vi "nanocal -- nuclear schottky goodness V3.vi"(7 "weighting strategy":T1, 8 "dz/dω IN (V)":cdb[](array[numeric])=[1.7183506006211996e-05+0.0i, 1.7124360968751133e-05+0.0i, 1.7049104347380084e-05+0.0i, 1.700437896335042e-05+0.0i, 1.6984579723285106e-05+0.0i, 1.702277369054923e-05+0.0i, 1.713094025845651e-05+0.0i, 1.734249707866828e-05+0.0i, 1.768320429215342e-05+0.0i, 1.8195281152538477e-05+0.0i, 1.8917228661806973e-05+0.0i, 1.9897834564883332e-05+0.0i, 2.154104046962704e-05+0.0i, 2.3247799321765792e-05+0.0i, 2.5364678450551808e-05+0.0i, 2.8645788781885885e-05+0.0i, 3.204749554800641e-05+0.0i, 3.783559691555022e-05+0.0i, 4.245015867332296e-05+0.0i, 4.909131821431355e-05+0.0i, 5.511821898441184e-05+0.0i, 6.178843506022867e-05+0.0i, 7.1079604965352e-05+0.0i, 7.922304381453334e-05+0.0i, 8.814778883893872e-05+0.0i, 9.806709148886077e-05+0.0i, 0.00011119043245647465+0.0i, 0.00012253184919712196+0.0i, 0.00013777724317049346+0.0i, 0.0001508081004573332+0.0i, 0.00016547294918783876+0.0i, 0.00018003847596605868+0.0i, 0.00019518361086534857+0.0i, 0.00021134179818259658+0.0i, 0.0002372041782935464+0.0i, 0.00025518143132024254+0.0i, 0.0002835129702467886+0.0i, 0.0003060118087631287+0.0i, 0.00032860772064336976+0.0i, 0.0003492674091322389+0.0i, 0.00037498324855458583+0.0i, 0.00040021078021115026+0.0i, 0.00041969942568205823+0.0i, 0.00044367338947118773+0.0i, 0.0004634793607238068+0.0i, 0.00047921028781215815+0.0i, 0.0004880906353641744+0.0i, 0.0004932212623741357+0.0i, 0.000491476456593048+0.0i, 0.000480893803992059+0.0i, 0.0004535995818650303+0.0i, 0.000417087772881063+0.0i, 0.0003564148692854789+0.0i, 0.0003049201646356487+0.0i, 0.00021260191240459413+0.0i, 0.00011714858948470126+0.0i, 1.675457544365132e-05+0.0i, -6.8674075405897e-05+0.0i, -0.000156473047607305+0.0i, -0.00026709373934749337+0.0i, -0.0003544271565676041+0.0i, -0.00047937600197311275+0.0i, -0.0006086290582260493+0.0i, -0.0007031877411848573+0.0i, -0.0007564526901441745+0.0i, -0.000802489180995596+0.0i, -0.0008414596018105983+0.0i, -0.0008809346482248761+0.0i, -0.0009073902840241921+0.0i, -0.0009264953054508651+0.0i, -0.0009405659412141811+0.0i, -0.000951649722530156+0.0i, -0.0009557485581057351+0.0i, -0.0009558464741053665+0.0i, -0.0009509110176922098+0.0i, -0.0009411315169847015+0.0i, -0.0009303400913929496+0.0i, -0.0009171113529290538+0.0i, -0.0009022111527275027+0.0i, -0.0008813746494947608+0.0i, -0.0008581837971946129+0.0i, -0.0008372063466683705+0.0i, -0.0008165626610594428+0.0i, -0.0007901155435838691+0.0i, -0.0007682834352800848+0.0i, -0.000746231015527196+0.0i, -0.0007238798463130141+0.0i, -0.0007015567569177018+0.0i, -0.000679301954671598+0.0i, -0.0006572001413831251+0.0i, -0.000629855254567978+0.0i, -0.0006083942229188815+0.0i, -0.0005768631156754208+0.0i, -0.0005562177438951648+0.0i, -0.0005359092039599222+0.0i, -0.0005145186443378148+0.0i, -0.0004951602053444319+0.0i, -0.00047624970229075174+0.0i, -0.0004577401041527736+0.0i, -0.00043519037796120065+0.0i], 9 "Voltage IN (V)":cdb[](array[numeric])=[1.7183506006211996e-05+0.0i, 1.7124360968751133e-05+0.0i, 1.7049104347380084e-05+0.0i, 1.700437896335042e-05+0.0i, 1.6984579723285106e-05+0.0i, 1.702277369054923e-05+0.0i, 1.713094025845651e-05+0.0i, 1.734249707866828e-05+0.0i, 1.768320429215342e-05+0.0i, 1.8195281152538477e-05+0.0i, 1.8917228661806973e-05+0.0i, 1.9897834564883332e-05+0.0i, 2.154104046962704e-05+0.0i, 2.3247799321765792e-05+0.0i, 2.5364678450551808e-05+0.0i, 2.8645788781885885e-05+0.0i, 3.204749554800641e-05+0.0i, 3.783559691555022e-05+0.0i, 4.245015867332296e-05+0.0i, 4.909131821431355e-05+0.0i, 5.511821898441184e-05+0.0i, 6.178843506022867e-05+0.0i, 7.1079604965352e-05+0.0i, 7.922304381453334e-05+0.0i, 8.814778883893872e-05+0.0i, 9.806709148886077e-05+0.0i, 0.00011119043245647465+0.0i, 0.00012253184919712196+0.0i, 0.00013777724317049346+0.0i, 0.0001508081004573332+0.0i, 0.00016547294918783876+0.0i, 0.00018003847596605868+0.0i, 0.00019518361086534857+0.0i, 0.00021134179818259658+0.0i, 0.0002372041782935464+0.0i, 0.00025518143132024254+0.0i, 0.0002835129702467886+0.0i, 0.0003060118087631287+0.0i, 0.00032860772064336976+0.0i, 0.0003492674091322389+0.0i, 0.00037498324855458583+0.0i, 0.00040021078021115026+0.0i, 0.00041969942568205823+0.0i, 0.00044367338947118773+0.0i, 0.0004634793607238068+0.0i, 0.00047921028781215815+0.0i, 0.0004880906353641744+0.0i, 0.0004932212623741357+0.0i, 0.000491476456593048+0.0i, 0.000480893803992059+0.0i, 0.0004535995818650303+0.0i, 0.000417087772881063+0.0i, 0.0003564148692854789+0.0i, 0.0003049201646356487+0.0i, 0.00021260191240459413+0.0i, 0.00011714858948470126+0.0i, 1.675457544365132e-05+0.0i, -6.8674075405897e-05+0.0i, -0.000156473047607305+0.0i, -0.00026709373934749337+0.0i, -0.0003544271565676041+0.0i, -0.00047937600197311275+0.0i, -0.0006086290582260493+0.0i, -0.0007031877411848573+0.0i, -0.0007564526901441745+0.0i, -0.000802489180995596+0.0i, -0.0008414596018105983+0.0i, -0.0008809346482248761+0.0i, -0.0009073902840241921+0.0i, -0.0009264953054508651+0.0i, -0.0009405659412141811+0.0i, -0.000951649722530156+0.0i, -0.0009557485581057351+0.0i, -0.0009558464741053665+0.0i, -0.0009509110176922098+0.0i, -0.0009411315169847015+0.0i, -0.0009303400913929496+0.0i, -0.0009171113529290538+0.0i, -0.0009022111527275027+0.0i, -0.0008813746494947608+0.0i, -0.0008581837971946129+0.0i, -0.0008372063466683705+0.0i, -0.0008165626610594428+0.0i, -0.0007901155435838691+0.0i, -0.0007682834352800848+0.0i, -0.000746231015527196+0.0i, -0.0007238798463130141+0.0i, -0.0007015567569177018+0.0i, -0.000679301954671598+0.0i, -0.0006572001413831251+0.0i, -0.000629855254567978+0.0i, -0.0006083942229188815+0.0i, -0.0005768631156754208+0.0i, -0.0005562177438951648+0.0i, -0.0005359092039599222+0.0i, -0.0005145186443378148+0.0i, -0.0004951602053444319+0.0i, -0.00047624970229075174+0.0i, -0.0004577401041527736+0.0i, -0.00043519037796120065+0.0i], 10 "ω (rad/sec)":dbl[](array[numeric])=[32012.991918577427, 32390.261658505893, 32466.39798177853, 32499.14340521798, 32517.39286113775, 32529.046092051318, 32537.14525712326, 32543.111142615544, 32547.696343954158, 32551.33675949651, 32554.302325209504, 32556.769142360055, 32558.856995237307, 32560.650202739795, 32562.209843476354, 32563.58125099723, 32564.7987833122, 32565.88895894197, 32566.872575330308, 32567.766175404246, 32568.583086316496, 32569.334166794306, 32570.02835688638, 32570.673085530187, 32571.274580490695, 32571.838104118455, 32572.36813539066, 32572.868514009202, 32573.342552524307, 32573.793126289274, 32574.222746575288, 32574.633618125405, 32575.027687968828, 32575.40668442971, 32575.772149741057, 32576.12546690325, 32576.467883345118, 32576.800529469096, 32577.124435064776, 32577.440543590797, 32577.749724325146, 32578.052781957467, 32578.35046682089, 32578.643482565894, 32578.932492128843, 32579.218126471686, 32579.500987779396, 32579.781656707495, 32580.06069600583, 32580.338656060805, 32580.616078519142, 32580.89350097748, 32581.171461032456, 32581.45050033079, 32581.73116925889, 32582.0140305666, 32582.29966469628, 32582.58867447239, 32582.88169000423, 32583.179375080817, 32583.48243271314, 32583.791613234323, 32584.10772197351, 32584.43162756919, 32584.764273480003, 32585.106690135035, 32585.460007297228, 32585.825472395412, 32586.204468856296, 32586.59853891288, 32587.009410462997, 32587.439030535847, 32587.889604513977, 32588.363642815923, 32588.86402143446, 32589.39405291983, 32589.957576334426, 32590.559071508098, 32591.203800151903, 32591.897990030815, 32592.64907072179, 32593.46598163404, 32594.359581707977, 32595.343197883154, 32596.433373726086, 32597.650906041054, 32599.022313348767, 32600.58195429849, 32602.375161800977, 32604.46301467823, 32606.929831615616, 32609.895397541775, 32613.535812870963, 32618.12101442274, 32624.086899701866, 32632.186064986967, 32643.839295900536, 32662.088751820305, 32694.834175046595, 32770.97049853239], 11 "parameters":dbl[](array[numeric])=[-0.0007412078466363201, -0.0004027798896083045, -0.019859061457473383, -0.00809909374498405, -0.08771864860021968, -0.6888815311338856]) -> (0 "R norm":dbl=-1.0, 1 "G":dbl=-1.0, 2 "derivatives":dbl[](array[numeric])=[-0.0007412078466363201, -0.0004027798896083045, -0.019859061457473383, -0.00809909374498405, -0.08771864860021968, -0.6888815311338856], 3 "parameters OUT":dbl[](array[numeric])=[-0.0007412078466363201, -0.0004027798896083045, -0.019859061457473383, -0.00809909374498405, -0.08771864860021968, -0.6888815311338856], 4 "R(ω) out":cdb[](array[numeric])=[1.7183506006211996e-05+0.0i, 1.7124360968751133e-05+0.0i, 1.7049104347380084e-05+0.0i, 1.700437896335042e-05+0.0i, 1.6984579723285106e-05+0.0i, 1.702277369054923e-05+0.0i, 1.713094025845651e-05+0.0i, 1.734249707866828e-05+0.0i, 1.768320429215342e-05+0.0i, 1.8195281152538477e-05+0.0i, 1.8917228661806973e-05+0.0i, 1.9897834564883332e-05+0.0i, 2.154104046962704e-05+0.0i, 2.3247799321765792e-05+0.0i, 2.5364678450551808e-05+0.0i, 2.8645788781885885e-05+0.0i, 3.204749554800641e-05+0.0i, 3.783559691555022e-05+0.0i, 4.245015867332296e-05+0.0i, 4.909131821431355e-05+0.0i, 5.511821898441184e-05+0.0i, 6.178843506022867e-05+0.0i, 7.1079604965352e-05+0.0i, 7.922304381453334e-05+0.0i, 8.814778883893872e-05+0.0i, 9.806709148886077e-05+0.0i, 0.00011119043245647465+0.0i, 0.00012253184919712196+0.0i, 0.00013777724317049346+0.0i, 0.0001508081004573332+0.0i, 0.00016547294918783876+0.0i, 0.00018003847596605868+0.0i, 0.00019518361086534857+0.0i, 0.00021134179818259658+0.0i, 0.0002372041782935464+0.0i, 0.00025518143132024254+0.0i, 0.0002835129702467886+0.0i, 0.0003060118087631287+0.0i, 0.00032860772064336976+0.0i, 0.0003492674091322389+0.0i, 0.00037498324855458583+0.0i, 0.00040021078021115026+0.0i, 0.00041969942568205823+0.0i, 0.00044367338947118773+0.0i, 0.0004634793607238068+0.0i, 0.00047921028781215815+0.0i, 0.0004880906353641744+0.0i, 0.0004932212623741357+0.0i, 0.000491476456593048+0.0i, 0.000480893803992059+0.0i, 0.0004535995818650303+0.0i, 0.000417087772881063+0.0i, 0.0003564148692854789+0.0i, 0.0003049201646356487+0.0i, 0.00021260191240459413+0.0i, 0.00011714858948470126+0.0i, 1.675457544365132e-05+0.0i, -6.8674075405897e-05+0.0i, -0.000156473047607305+0.0i, -0.00026709373934749337+0.0i, -0.0003544271565676041+0.0i, -0.00047937600197311275+0.0i, -0.0006086290582260493+0.0i, -0.0007031877411848573+0.0i, -0.0007564526901441745+0.0i, -0.000802489180995596+0.0i, -0.0008414596018105983+0.0i, -0.0008809346482248761+0.0i, -0.0009073902840241921+0.0i, -0.0009264953054508651+0.0i, -0.0009405659412141811+0.0i, -0.000951649722530156+0.0i, -0.0009557485581057351+0.0i, -0.0009558464741053665+0.0i, -0.0009509110176922098+0.0i, -0.0009411315169847015+0.0i, -0.0009303400913929496+0.0i, -0.0009171113529290538+0.0i, -0.0009022111527275027+0.0i, -0.0008813746494947608+0.0i, -0.0008581837971946129+0.0i, -0.0008372063466683705+0.0i, -0.0008165626610594428+0.0i, -0.0007901155435838691+0.0i, -0.0007682834352800848+0.0i, -0.000746231015527196+0.0i, -0.0007238798463130141+0.0i, -0.0007015567569177018+0.0i, -0.000679301954671598+0.0i, -0.0006572001413831251+0.0i, -0.000629855254567978+0.0i, -0.0006083942229188815+0.0i, -0.0005768631156754208+0.0i, -0.0005562177438951648+0.0i, -0.0005359092039599222+0.0i, -0.0005145186443378148+0.0i, -0.0004951602053444319+0.0i, -0.00047624970229075174+0.0i, -0.0004577401041527736+0.0i, -0.00043519037796120065+0.0i])   [LabVIEW 2020]
uses:
  nanocal-goodness-weighting-strategy.ctl
  3-lorentzian-heat-response action.ctl
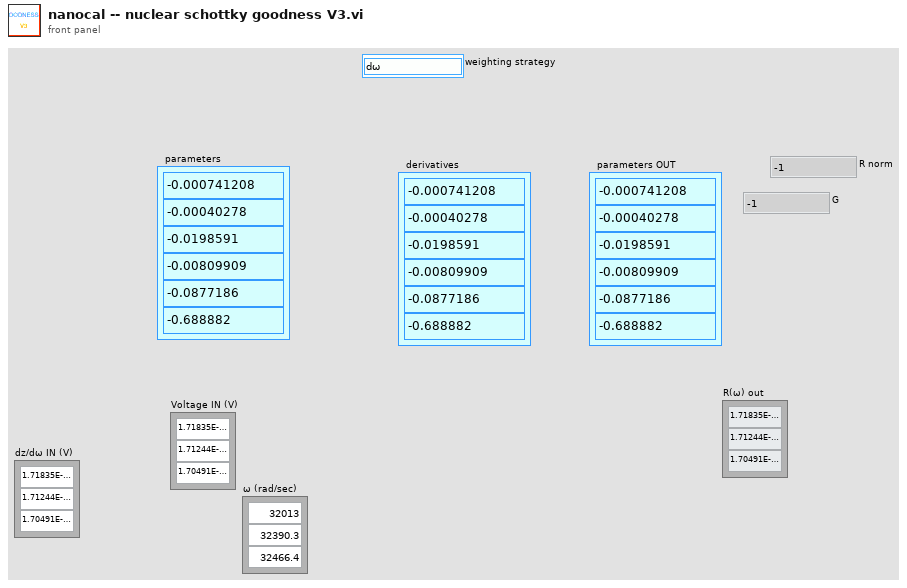
[diagram p1: front panel]
types:
  T1 = typedef "nanocal-goodness-weighting-strategy.ctl" = enum16{"dω", "dω √(|dz/dω|)", "dω |dz/dω|", "phase", "andreas", "sum"}
  T2 = typedef "3-lorentzian-heat-response action.ctl" = enum16{"calc R", "create string", "calc m1m2m3", "dζ", "dT1", "dτS", "dτN", "dτC", "d-all", "dκ0", "T(K)", "m1", "m2", "m3", "parse string", "θ (deg)", "B (T)", "onlygrads", "newton", "create emty string"}
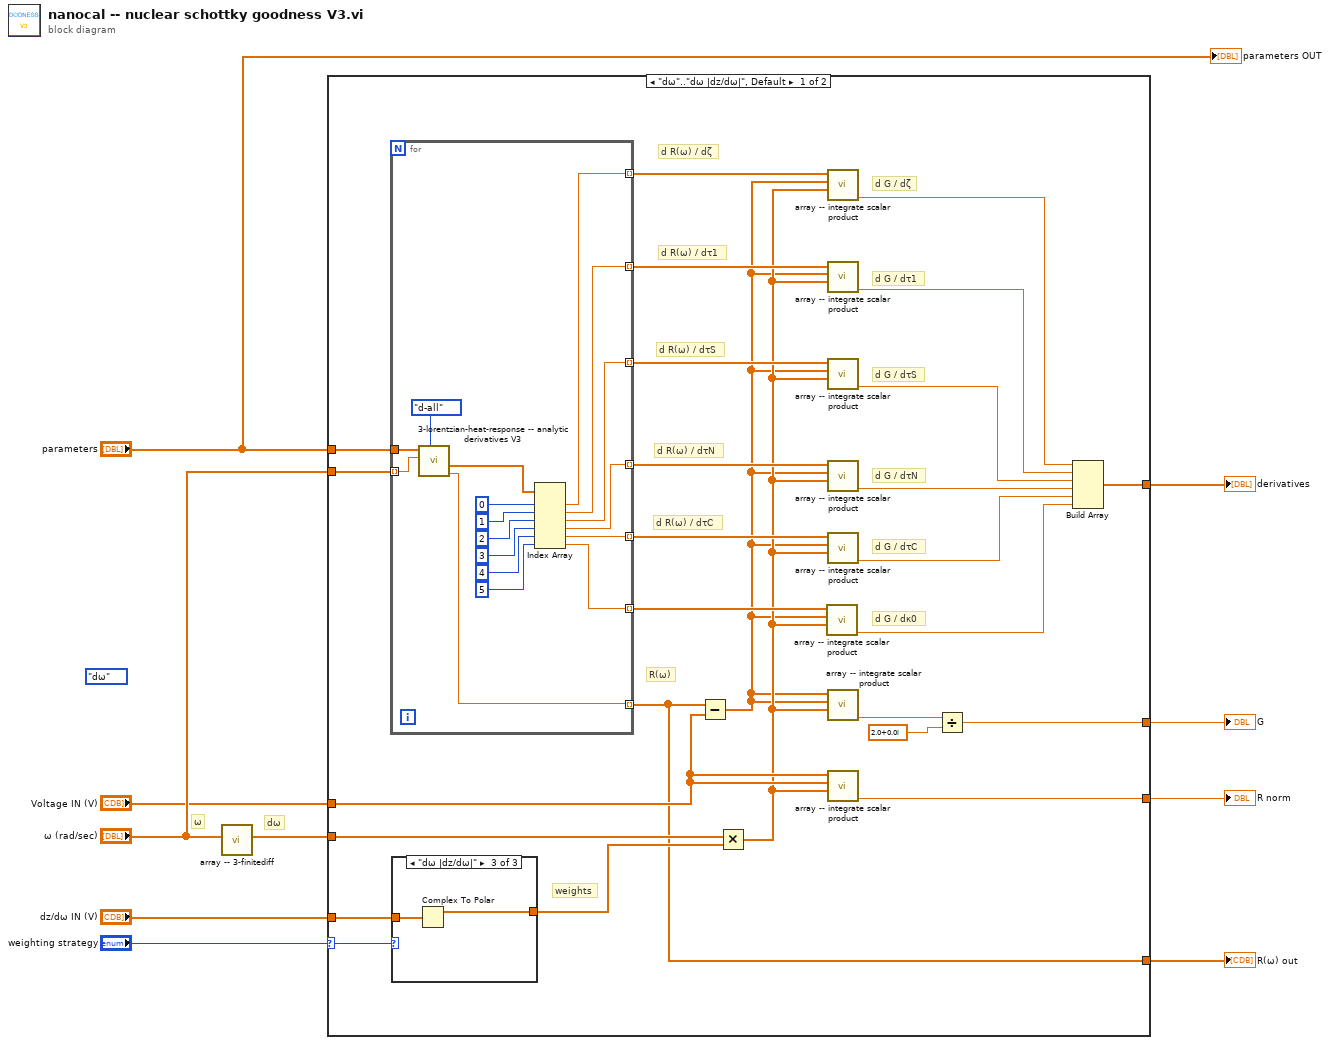
[diagram p0: block diagram]
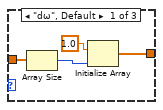
[diagram p2: hidden frame]
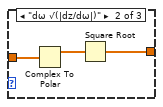
[diagram p3: hidden frame]
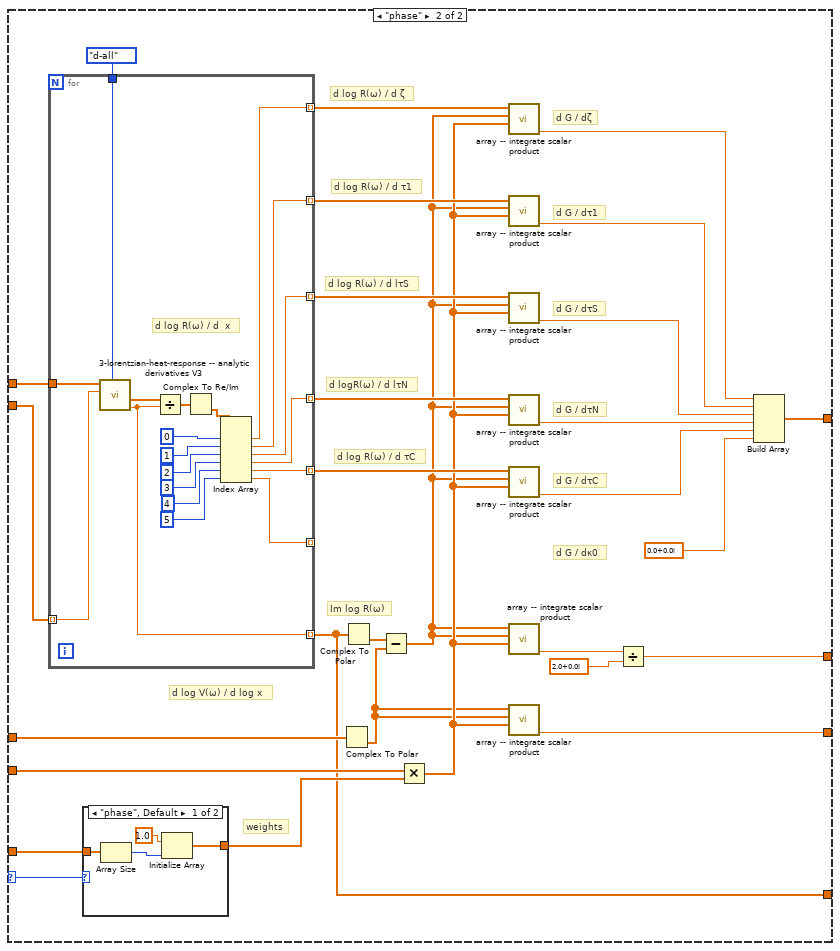
[diagram p4: hidden frame]
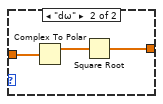
[diagram p5: hidden frame]
diagram:
  (unwired) nanocal-goodness-weighting-strategy."dω" ("action")
  # "ω"
  # "dω"
  n1 = call "array -- 3-finitediff.vi"("ω (rad/sec)"="ω (rad/sec)") -> ("dω (rad/sec)"=w10:cdb[])  [unwired: 10 in]
  n2 = case shown="\"dω\"..\"dω |dz/dω|\", Default" "weighting strategy" {
    selector: "weighting strategy" -> [w12 w72]
    tunnel: w10 -> [w30 w85]
    tunnel: "ω (rad/sec)" -> [w29 w70]
    tunnel: "Voltage IN (V)" -> [w28 w68]
    tunnel: "dz/dω IN (V)" -> [w23 w69]
    tunnel: [w17 w77] -> w6
    tunnel: [w16 w76] -> w5
    tunnel: [w15 w75] -> w4
    tunnel: "parameters" -> [w13 w73]
    tunnel: [w11 w64] -> w1
    frame "dω".."dω |dz/dω|", Default {
      # "weights"
      # "d G / dκ0"
      # "d G / dτC"
      # "d G / dτN"
      # "d G / dτS"
      # "d G / dτ1"
      # "d G / dζ"
      # "d R(ω) / dτC"
      # "d R(ω) / dτN"
      # "d R(ω) / dτS"
      # "d R(ω) / dτ1"
      # "d R(ω) / dζ"
      # "R(ω)"
      n3 = for {
        tunnel: w29 -> [w62] mode=indexing
        tunnel: [w48] -> w11 mode=indexing
        tunnel: [w54] -> w37 mode=indexing
        tunnel: [w53] -> w36 mode=indexing
        tunnel: [w52] -> w35 mode=indexing
        tunnel: [w51] -> w34 mode=indexing
        tunnel: [w50] -> w33 mode=indexing
        tunnel: [w49] -> w32 mode=indexing
        tunnel: w13 -> [w63]
        n4 = call "3-lorentzian-heat-response -- analytic derivatives V3.vi"("action"=3-lorentzian-heat-response_action."d-all", "ω (rad/sec)"=w62, "parameters"=w63) -> ("R(ω)"=w48:cdb, "derivatives"=w55:cdb[])  [unwired: 5 in, 2 out]
        n5 = Index Array(array=w55, index #1=0 ("index"), index #2=1 ("index"), index #3=2 ("index"), index #4=3 ("index"), index #5=4 ("index"), index #6=5 ("index")) -> (element #1=w54:cdb, element #2=w53:cdb, element #3=w52:cdb, element #4=w51:cdb, element #5=w50:cdb, element #6=w49:cdb)
      }
      n6 = case shown="\"dω |dz/dω|\"" w12 {
        tunnel: [w38 w42 w45] -> w25
        tunnel: w23 -> [w40 w44 w46]
        frame "dω", Default {
          n7 = Array Size(array=w40) -> (size(s)=w41:i32)
          n8 = Initialize Array(1.0 ("element"), w41) -> (w38:dbl[])
        }
        frame "dω √(|dz/dω|)" {
          n9 = Complex To Polar(r * e^(i*theta)=w44) -> (r=w43:dbl[])  [unwired: 1 out]
          n10 = Square Root(x=w43) -> (sqrt(x)=w42:dbl[])
        }
        frame "dω |dz/dω|" {
          n11 = Complex To Polar(r * e^(i*theta)=w46) -> (r=w45:dbl[])  [unwired: 1 out]
        }
      }
      n12 = Subtract(x=w11, y=w28) -> (x-y=w24:cdb[])
      n13 = Multiply(x=w30, y=w25) -> (x*y=w27:cdb[])
      n14 = call "array -- integrate scalar product.vi"("dω"=w27, "B"=w24, "A"=w32) -> ("total"=w18:cdb)  [unwired: 7 in, 1 out]
      n15 = call "array -- integrate scalar product.vi"("dω"=w27, "B"=w24, "A"=w37) -> ("total"=w14:cdb)  [unwired: 7 in, 1 out]
      n16 = call "array -- integrate scalar product.vi"("dω"=w27, "B"=w24, "A"=w36) -> ("total"=w22:cdb)  [unwired: 7 in, 1 out]
      n17 = call "array -- integrate scalar product.vi"("dω"=w27, "B"=w24, "A"=w35) -> ("total"=w21:cdb)  [unwired: 7 in, 1 out]
      n18 = call "array -- integrate scalar product.vi"("dω"=w27, "B"=w24, "A"=w34) -> ("total"=w20:cdb)  [unwired: 7 in, 1 out]
      n19 = call "array -- integrate scalar product.vi"("dω"=w27, "B"=w24, "A"=w33) -> ("total"=w19:cdb)  [unwired: 7 in, 1 out]
      n20 = call "array -- integrate scalar product.vi"("dω"=w27, "B"=w24, "A"=w24) -> ("total"=w26:cdb)  [unwired: 7 in, 1 out]
      n21 = call "array -- integrate scalar product.vi"("dω"=w27, "B"=w28, "A"=w28) -> ("total"=w16:cdb)  [unwired: 7 in, 1 out]
      n22 = Divide(x=w26, y=cdb 2.0+0.0i) -> (x/y=w17:cdb)
      n23 = Build Array(w14, w22, w21, w20, w19, w18) -> (w15:cdb[])
    }
    frame "phase" {
      # "d log V(ω) / d log x"
      # "weights"
      # "d G / dκ0"
      # "d G / dτC"
      # "d G / dτN"
      # "d G / dτS"
      # "d G / dτ1"
      # "d G / dζ"
      # "d log R(ω) / d τC"
      # "d logR(ω) / d lτN"
      # "d log R(ω) / d lτS"
      # "d log R(ω) / d τ1"
      # "d log R(ω) / d ζ"
      # "Im log R(ω)"
      n24 = for {
        tunnel: 3-lorentzian-heat-response_action."d-all" ("action") -> [w117]
        tunnel: w70 -> [w116] mode=indexing
        tunnel: [w109] -> w91 mode=indexing
        tunnel: [w108] -> w90 mode=indexing
        tunnel: [w107] -> w89 mode=indexing
        tunnel: [w106] -> w88 mode=indexing
        tunnel: [w105] -> w87 mode=indexing
        tunnel: [w104] -> _ mode=indexing
        tunnel: w73 -> [w118]
        tunnel: [w100] -> w64 mode=indexing
        # "d log R(ω) / d  x"
        n25 = call "3-lorentzian-heat-response -- analytic derivatives V3.vi"("action"=w117, "ω (rad/sec)"=w116, "parameters"=w118) -> ("R(ω)"=w100:cdb, "derivatives"=w101:cdb[])  [unwired: 5 in, 2 out]
        n26 = Divide(x=w101, y=w100) -> (x/y=w103:cdb[])
        n27 = Complex To Re/Im(x + iy=w103) -> (y=w102:dbl[])  [unwired: 1 out]
        n28 = Index Array(array=w102, index #1=0 ("index"), index #2=1 ("index"), index #3=2 ("index"), index #4=3 ("index"), index #5=4 ("index"), index #6=5 ("index")) -> (element #1=w109:dbl, element #2=w108:dbl, element #3=w107:dbl, element #4=w106:dbl, element #5=w105:dbl, element #6=w104:dbl)
      }
      n29 = case shown="\"phase\", Default" w72 {
        tunnel: [w93 w97] -> w71
        tunnel: w69 -> [w95 w99]
        frame "phase", Default {
          n30 = Array Size(array=w95) -> (size(s)=w96:i32)
          n31 = Initialize Array(1.0 ("element"), w96) -> (w93:dbl[])
        }
        frame "dω" {
          n32 = Complex To Polar(r * e^(i*theta)=w99) -> (r=w98:dbl[])  [unwired: 1 out]
          n33 = Square Root(x=w98) -> (sqrt(x)=w97:dbl[])
        }
      }
      n34 = Complex To Polar(r * e^(i*theta)=w68) -> (theta=w67:dbl[])  [unwired: 1 out]
      n35 = Complex To Polar(r * e^(i*theta)=w64) -> (theta=w65:dbl[])  [unwired: 1 out]
      n36 = Subtract(x=w65, y=w67) -> (x-y=w82:dbl[])
      n37 = Multiply(x=w85, y=w71) -> (x*y=w84:cdb[])
      n38 = call "array -- integrate scalar product.vi"("dω"=w84, "B"=w82, "A"=w91) -> ("total"=w74:cdb)  [unwired: 7 in, 1 out]
      n39 = call "array -- integrate scalar product.vi"("dω"=w84, "B"=w82, "A"=w90) -> ("total"=w81:cdb)  [unwired: 7 in, 1 out]
      n40 = call "array -- integrate scalar product.vi"("dω"=w84, "B"=w82, "A"=w89) -> ("total"=w80:cdb)  [unwired: 7 in, 1 out]
      n41 = call "array -- integrate scalar product.vi"("dω"=w84, "B"=w82, "A"=w88) -> ("total"=w79:cdb)  [unwired: 7 in, 1 out]
      n42 = call "array -- integrate scalar product.vi"("dω"=w84, "B"=w82, "A"=w87) -> ("total"=w78:cdb)  [unwired: 7 in, 1 out]
      n43 = call "array -- integrate scalar product.vi"("dω"=w84, "B"=w82, "A"=w82) -> ("total"=w83:cdb)  [unwired: 7 in, 1 out]
      n44 = call "array -- integrate scalar product.vi"("dω"=w84, "B"=w67, "A"=w67) -> ("total"=w76:cdb)  [unwired: 7 in, 1 out]
      n45 = Divide(x=w83, y=cdb 2.0+0.0i) -> (x/y=w77:cdb)
      n46 = Build Array(w74, w81, w80, w79, w78, cdb 0.0+0.0i ("element")) -> (w75:cdb[])
    }
  }
  "G" <- w6
  "derivatives" <- w4
  "R norm" <- w5
  "R(ω) out" <- w1
  "parameters OUT" <- "parameters"
